vi "Calibrate Axis Command.vi"(8 "Error In":errorcluster, 9 "Axis Enum":T1=enum."Z-axis", 10 "Duty Cycle (%)":dbl) -> (0 "Error Out":errorcluster, 1 "Axis Enum out":T1=enum."Z-axis", 2 "Calib. Duty Cycle":dbl)   [LabVIEW 2013]
doc: "This sub-VI scales a desired duty cycle (-100, 100) to the range of applicable duty cycles for the given axis.\nApplicable duty cycle range is based on the dead-zone calibration data stored in Axis_calibration_cluster.vi.\nNote: linear scaling is applied."
uses:
  Controls/table_axis_enum.ctl
  Globals/Axis_calibration_cluster.vi
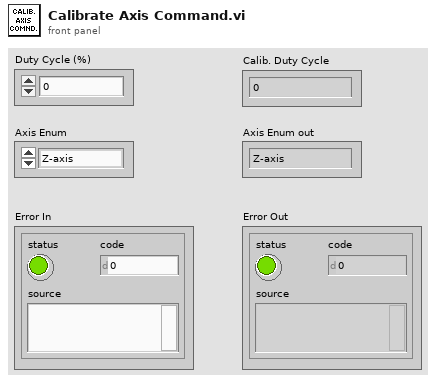
[diagram p1: front panel]
types:
  T1 = typedef "table_axis_enum.ctl" = enum16{"X-axis", "Y-axis", "Z-axis", "W-axis"}
  T2 = cluster{"Min neg. X":dbl, "Max neg. X":dbl, "Min pos. X":dbl, "Max pos. X":dbl, "Min neg. Y":dbl, "Max neg. Y":dbl, "Min pos. Y":dbl, "Max pos. Y":dbl, "Min neg. Z":dbl, "Max neg. Z":dbl, "Min pos. Z":dbl, "Max pos. Z":dbl, "Min neg. W":dbl, "Max neg. W":dbl, "Min pos. W":dbl, "Max pos. W":dbl}
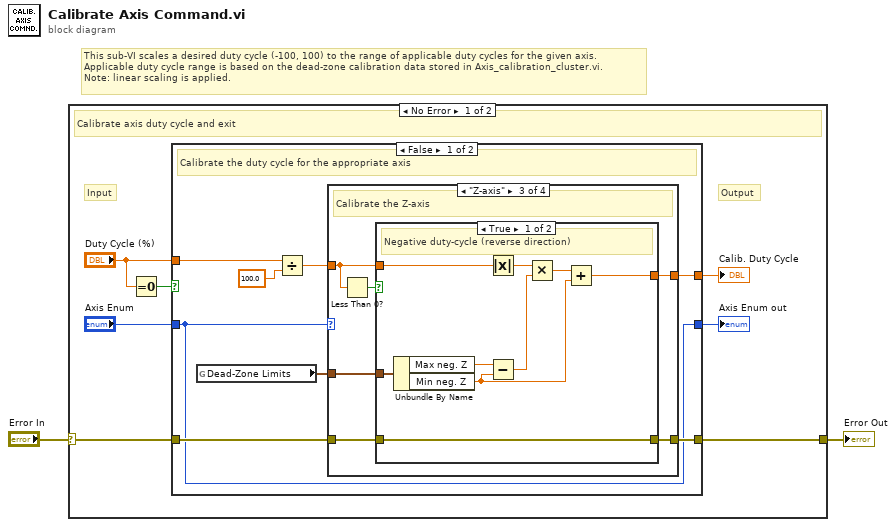
[diagram p0: block diagram]
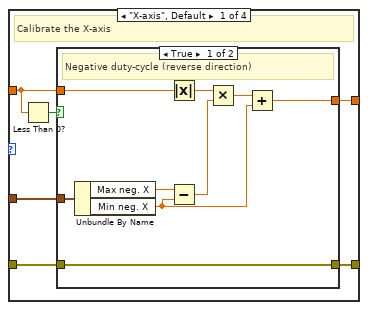
[diagram p2: hidden frame]
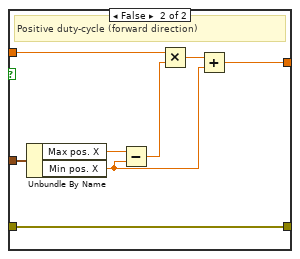
[diagram p3: hidden frame]
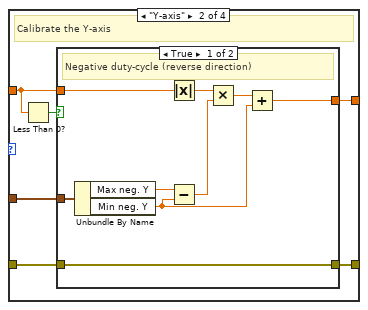
[diagram p4: hidden frame]
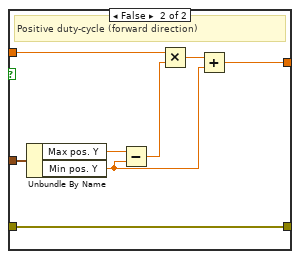
[diagram p5: hidden frame]
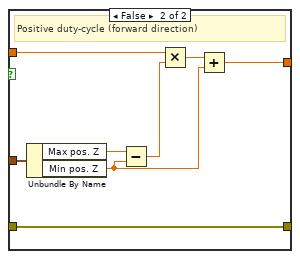
[diagram p6: hidden frame]
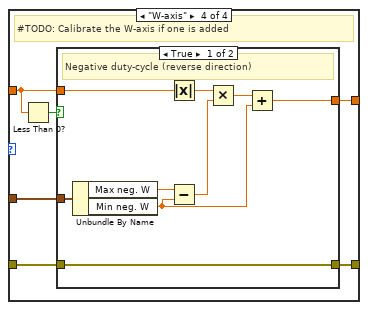
[diagram p7: hidden frame]
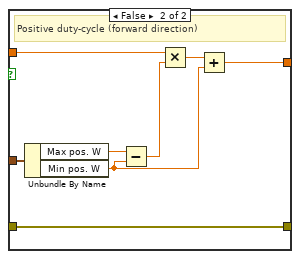
[diagram p8: hidden frame]
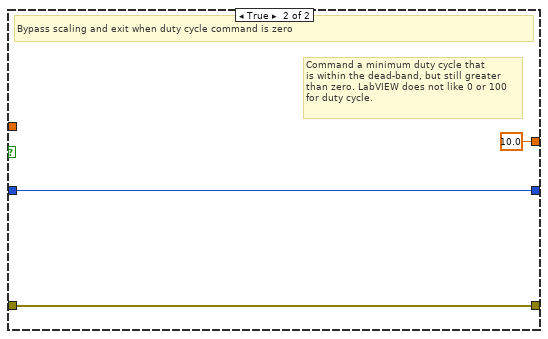
[diagram p9: hidden frame]
diagram:
  # "This sub-VI scales a desired duty cycle (-100, 100) to the range of applicable duty cycles for the given axis.\nApplicable duty cycle range is based on the dead-zone calibration data stored in Axis_calibration_cluster.vi.\nNote: linear scaling is applied."
  n1 = case shown="No Error" "Error In" {
    selector: "Error In" -> [w9 w113]
    tunnel: [w8 w113] -> w1
    frame No Error {
      # "Input"
      # "Output"
      # "Calibrate axis duty cycle and exit"
      n2 = Equal To 0?(x="Duty Cycle (%)") -> (x = 0?=w6:bool)
      n3 = case shown="False" w6 {
        tunnel: w9 -> [w16 w112]
        tunnel: [w15 w112] -> w8
        tunnel: "Duty Cycle (%)" -> [w14 _]
        tunnel: [w11 10.0] -> w7
        tunnel: "Axis Enum" -> [w10 w110]
        tunnel: [w10 w110] -> w3
        frame False {
          # "Calibrate the duty cycle for the appropriate axis"
          n4 = global read "Axis_calibration_cluster.vi" "Dead-Zone Limits"() -> (w17:T2)
          n5 = Divide(x=w14, y=100.0) -> (x/y=w12:dbl)
          n6 = case shown="\"Z-axis\"" w10 {
            tunnel: w16 -> [w23 w46 w69 w92]
            tunnel: [w22 w45 w68 w91] -> w15
            tunnel: w17 -> [w19 w42 w65 w88]
            tunnel: w12 -> [w20 w43 w66 w89]
            tunnel: [w18 w41 w64 w87] -> w11
            frame "X-axis", Default {
              # "Calibrate the X-axis"
              n7 = Less Than 0?(x=w20) -> (x < 0?=w21:bool)
              n8 = case shown="True" w21 {
                tunnel: w23 -> [w32 w40]
                tunnel: [w32 w40] -> w22
                tunnel: w20 -> [w29 w37]
                tunnel: w19 -> [w31 w39]
                tunnel: [w25 w33] -> w18
                frame True {
                  # "Negative duty-cycle (reverse direction)"
                  n9 = Unbundle By Name(w31) -> ("Max neg. X"=w30:dbl, "Min neg. X"=w26:dbl)
                  n10 = Absolute Value(x=w29) -> (abs(x)=w24:dbl)
                  n11 = Subtract(x=w30, y=w26) -> (x-y=w28:dbl)
                  n12 = Multiply(x=w24, y=w28) -> (x*y=w27:dbl)
                  n13 = Add(x=w27, y=w26) -> (x+y=w25:dbl)
                }
                frame False {
                  # "Positive duty-cycle (forward direction)"
                  n14 = Unbundle By Name(w39) -> ("Max pos. X"=w38:dbl, "Min pos. X"=w34:dbl)
                  n15 = Subtract(x=w38, y=w34) -> (x-y=w36:dbl)
                  n16 = Multiply(x=w37, y=w36) -> (x*y=w35:dbl)
                  n17 = Add(x=w35, y=w34) -> (x+y=w33:dbl)
                }
              }
            }
            frame "Y-axis" {
              # "Calibrate the Y-axis"
              n18 = Less Than 0?(x=w43) -> (x < 0?=w44:bool)
              n19 = case shown="True" w44 {
                tunnel: w46 -> [w55 w63]
                tunnel: [w55 w63] -> w45
                tunnel: w43 -> [w52 w60]
                tunnel: w42 -> [w54 w62]
                tunnel: [w48 w56] -> w41
                frame True {
                  # "Negative duty-cycle (reverse direction)"
                  n20 = Unbundle By Name(w54) -> ("Max neg. Y"=w53:dbl, "Min neg. Y"=w49:dbl)
                  n21 = Absolute Value(x=w52) -> (abs(x)=w47:dbl)
                  n22 = Subtract(x=w53, y=w49) -> (x-y=w51:dbl)
                  n23 = Multiply(x=w47, y=w51) -> (x*y=w50:dbl)
                  n24 = Add(x=w50, y=w49) -> (x+y=w48:dbl)
                }
                frame False {
                  # "Positive duty-cycle (forward direction)"
                  n25 = Unbundle By Name(w62) -> ("Max pos. Y"=w61:dbl, "Min pos. Y"=w57:dbl)
                  n26 = Subtract(x=w61, y=w57) -> (x-y=w59:dbl)
                  n27 = Multiply(x=w60, y=w59) -> (x*y=w58:dbl)
                  n28 = Add(x=w58, y=w57) -> (x+y=w56:dbl)
                }
              }
            }
            frame "Z-axis" {
              # "Calibrate the Z-axis"
              n29 = Less Than 0?(x=w66) -> (x < 0?=w67:bool)
              n30 = case shown="True" w67 {
                tunnel: w69 -> [w78 w86]
                tunnel: [w78 w86] -> w68
                tunnel: w66 -> [w75 w83]
                tunnel: w65 -> [w77 w85]
                tunnel: [w71 w79] -> w64
                frame True {
                  # "Negative duty-cycle (reverse direction)"
                  n31 = Unbundle By Name(w77) -> ("Max neg. Z"=w76:dbl, "Min neg. Z"=w72:dbl)
                  n32 = Absolute Value(x=w75) -> (abs(x)=w70:dbl)
                  n33 = Subtract(x=w76, y=w72) -> (x-y=w74:dbl)
                  n34 = Multiply(x=w70, y=w74) -> (x*y=w73:dbl)
                  n35 = Add(x=w73, y=w72) -> (x+y=w71:dbl)
                }
                frame False {
                  # "Positive duty-cycle (forward direction)"
                  n36 = Unbundle By Name(w85) -> ("Max pos. Z"=w84:dbl, "Min pos. Z"=w80:dbl)
                  n37 = Subtract(x=w84, y=w80) -> (x-y=w82:dbl)
                  n38 = Multiply(x=w83, y=w82) -> (x*y=w81:dbl)
                  n39 = Add(x=w81, y=w80) -> (x+y=w79:dbl)
                }
              }
            }
            frame "W-axis" {
              # "#TODO: Calibrate the W-axis if one is added"
              n40 = Less Than 0?(x=w89) -> (x < 0?=w90:bool)
              n41 = case shown="True" w90 {
                tunnel: w92 -> [w101 w109]
                tunnel: [w101 w109] -> w91
                tunnel: w89 -> [w98 w106]
                tunnel: w88 -> [w100 w108]
                tunnel: [w94 w102] -> w87
                frame True {
                  # "Negative duty-cycle (reverse direction)"
                  n42 = Unbundle By Name(w100) -> ("Max neg. W"=w99:dbl, "Min neg. W"=w95:dbl)
                  n43 = Absolute Value(x=w98) -> (abs(x)=w93:dbl)
                  n44 = Subtract(x=w99, y=w95) -> (x-y=w97:dbl)
                  n45 = Multiply(x=w93, y=w97) -> (x*y=w96:dbl)
                  n46 = Add(x=w96, y=w95) -> (x+y=w94:dbl)
                }
                frame False {
                  # "Positive duty-cycle (forward direction)"
                  n47 = Unbundle By Name(w108) -> ("Max pos. W"=w107:dbl, "Min pos. W"=w103:dbl)
                  n48 = Subtract(x=w107, y=w103) -> (x-y=w105:dbl)
                  n49 = Multiply(x=w106, y=w105) -> (x*y=w104:dbl)
                  n50 = Add(x=w104, y=w103) -> (x+y=w102:dbl)
                }
              }
            }
          }
        }
        frame True {
          # "Command a minimum duty cycle that\nis within the dead-band, but still greater\nthan zero. LabVIEW does not like 0 or 100\nfor duty cycle."
          # "Bypass scaling and exit when duty cycle command is zero"
        }
      }
      "Calib. Duty Cycle" <- w7
      "Axis Enum out" <- w3
    }
    frame Error {
      # "Pass through and exit (do nothing)"
    }
  }
  "Error Out" <- w1
